vi "vision - Copy.vi"(0 "Image 3":T1(plugin-control)) -> ()   [LabVIEW 2018]
uses:
  Vision info.vi
panel:
  out "cir 2":cluster{"x":dbl, "y":dbl, "r":dbl}[](array[cluster])
  out "cir":cluster{"x":dbl, "y":dbl, "r":dbl}[](array[cluster])
  out "Circles 2":cluster{"x":dbl, "y":dbl, "r":dbl}[](array[cluster])
  out "cube found":bool
  out "Type":enum16{"Z", "I", "O", "S", "L", "J", "T", "N"}(ring)=enum."O"
  out "Discriptor":dbl[](array[numeric])
  out "Image 2":T1(plugin-control)
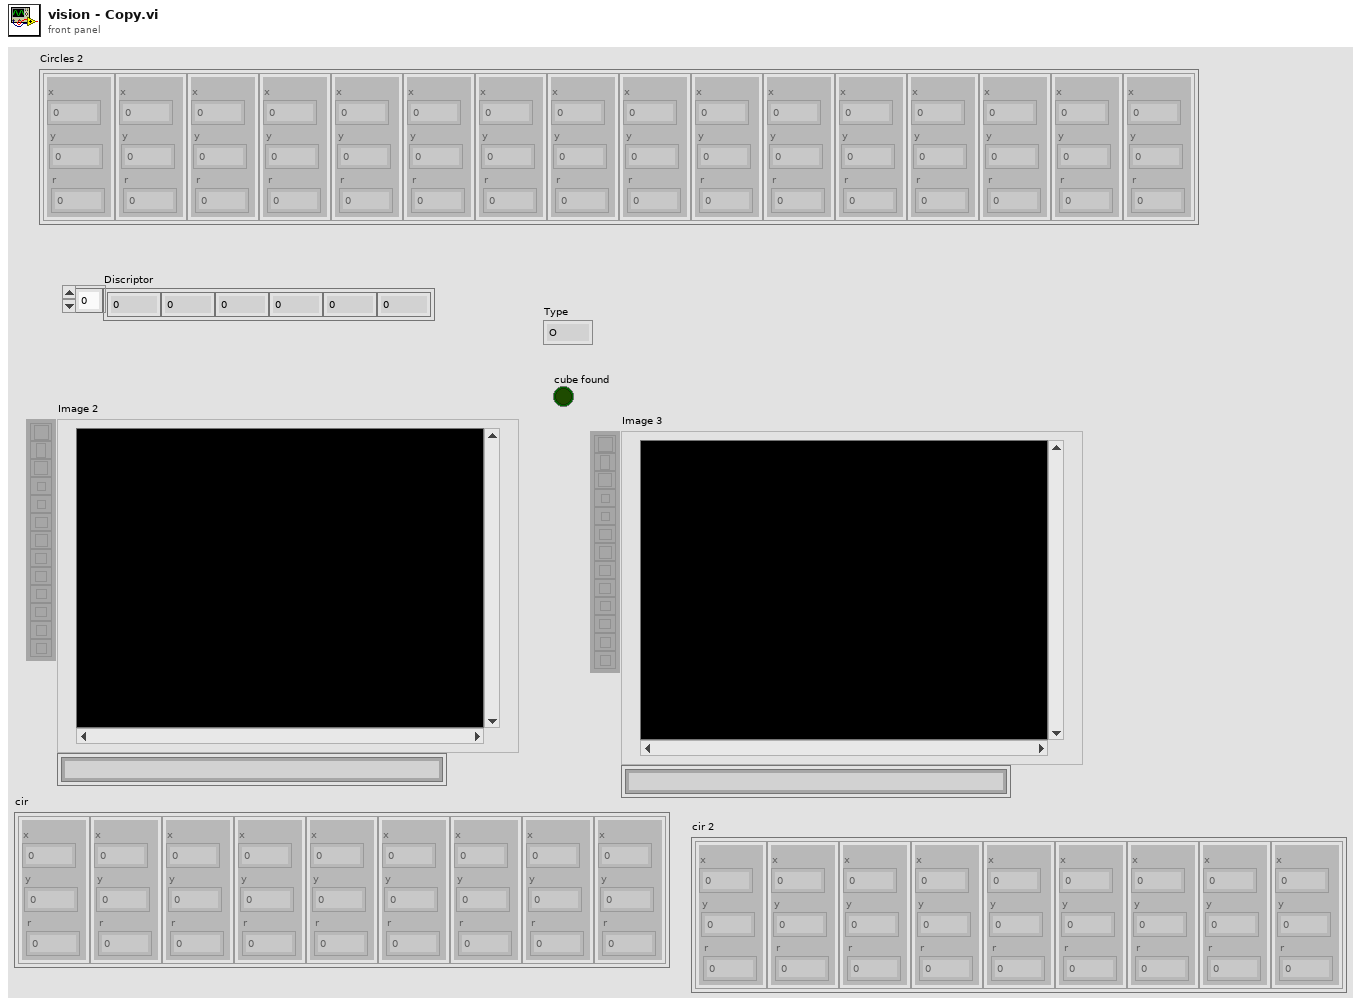
[diagram p1: front panel]
types:
  T1 = typedef "IMAQ Image.ctl" = refnum<image>
  T2 = cluster{"p1":cluster{"x":dbl, "y":dbl}, "p2":cluster{"x":dbl, "y":dbl}}
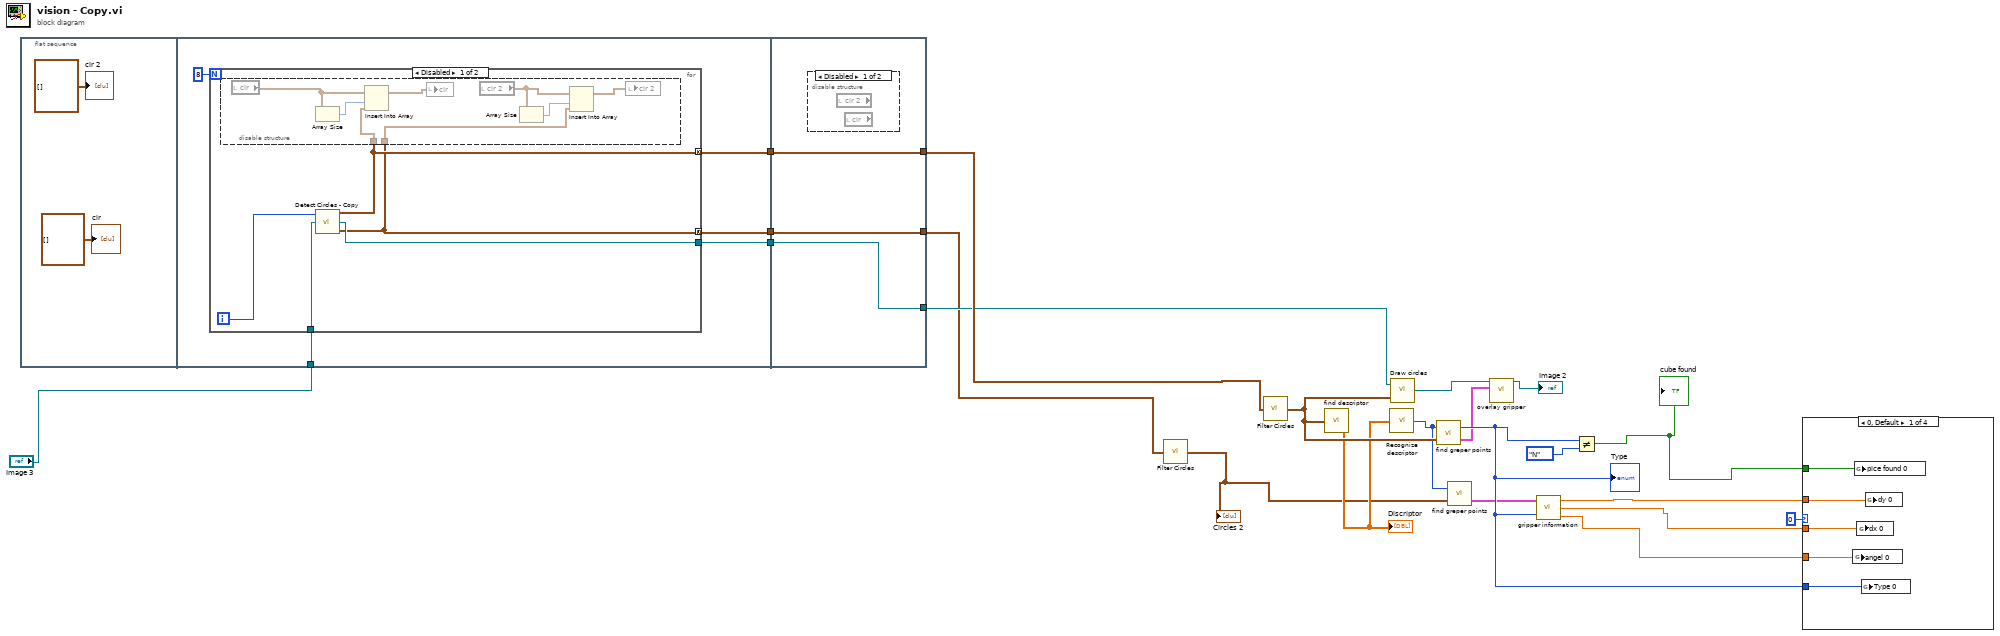
[diagram p0: block diagram]
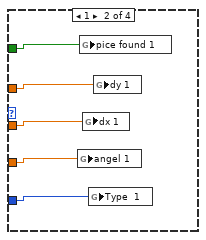
[diagram p4: hidden frame]
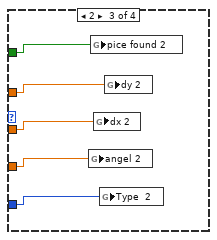
[diagram p5: hidden frame]
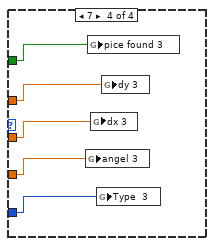
[diagram p6: hidden frame]
diagram:
  n1 = flat-sequence {
    tunnel: "Image 3" -> [w28]
    tunnel: [w27] -> w7
    tunnel: [w26] -> w4
    tunnel: [w25] -> w3
    tunnel: [w44] -> w8
    tunnel: [w43] -> w2
    tunnel: [w45] -> w5
    tunnel: w7 -> [w45]
    tunnel: w4 -> [w44]
    tunnel: w3 -> [w43]
    frame #0 {
      "cir" <- cluster{"x":dbl, "y":dbl, "r":dbl}[] [] ("cir")
      "cir 2" <- cluster{"x":dbl, "y":dbl, "r":dbl}[] [] ("cir")
    }
    frame #1 {
      n2 = for {
        N: 8 -> [_]
        tunnel: w28 -> [w33]
        tunnel: [w32] -> w27
        tunnel: [w31] -> w26 mode=concatenating
        tunnel: [w30] -> w25 mode=concatenating
        i -> [w34]
        n3 = call "Detect Circles - Copy.vi"("Image 3"=w33, "Color Plane"=w34) -> ("Circles 2"=w30:cluster{"x":dbl, "y":dbl, "r":dbl}[], "Image 4"=w32:T1, "Circles"=w31:cluster{"x":dbl, "y":dbl, "r":dbl}[])  [unwired: 1 in]
        n4 = disable-structure shown="Disabled" {
          disable-tunnel: w31 -> [w39 _]
          disable-tunnel: w30 -> [w36 _]
          frame Disabled {
            n5 = local read "cir"() -> (w41:cluster{"x":dbl, "y":dbl, "r":dbl}[])
            n6 = Array Size(array=w41) -> (size(s)=w40:i32)
            n7 = Insert Into Array(array=w41, index=w40, new element=w39) -> (w42:cluster{"x":dbl, "y":dbl, "r":dbl}[])
            n8 = local write "cir"(w42) -> ()
            n9 = local read "cir 2"() -> (w35:cluster{"x":dbl, "y":dbl, "r":dbl}[])
            n10 = Array Size(array=w35) -> (size(s)=w38:i32)
            n11 = Insert Into Array(array=w35, index=w38, new element=w36) -> (w37:cluster{"x":dbl, "y":dbl, "r":dbl}[])
            n12 = local write "cir 2"(w37) -> ()
          }
          frame Enabled {
          }
        }
      }
    }
    frame #2 {
      n13 = disable-structure shown="Disabled" {
        frame Disabled {
          n14 = local read "cir 2"() -> ()  [unwired: 1 out]
          n15 = local read "cir"() -> ()  [unwired: 1 out]
        }
        frame Enabled {
        }
      }
    }
  }
  n16 = call "Filter Circles.vi"("Circles"=w2) -> ("out"=w1:cluster{"x":dbl, "y":dbl, "r":dbl}[])
  "Circles 2" <- w1
  n17 = call "Filter Circles.vi"("Circles"=w8) -> ("out"=w17:cluster{"x":dbl, "y":dbl, "r":dbl}[])
  n18 = call "find descriptor.vi"("Circles"=w17) -> ("d"=w14:dbl[])
  "Discriptor" <- w14
  n19 = call "Recognize descriptor.vi"("Discriptor"=w14) -> ("Type"=w11:enum16{"Z", "I", "O", "S", "L", "J", "T", "N"})
  n20 = call "Draw circles .vi"("Circles"=w17, "Image 3"=w5) -> ("Refnum out"=w13:T1)
  n21 = call "find greper points.vi"("Circles"=w17, "Type  2"=w11) -> ("gripper"=w15:T2, "Type"=w22:enum16{"Z", "I", "O", "S", "L", "J", "T", "N"})
  "Type" <- w22
  n22 = call "find greper points.vi"("Circles"=w1, "Type  2"=w11) -> ("gripper"=w10:T2)  [unwired: 1 out]
  n23 = call "overlay gripper.vi"("gripper"=w15, "Refnum in"=w13) -> ("Refnum out"=→"Image 2":T1)  [unwired: 9 in]
  n24 = call "gripper information.vi"("gripper"=w10, "Type"=w22) -> ("dy"=w19:dbl, "dx"=w20:dbl, "Angel"=w21:dbl)
  n25 = Not Equal?(x=w22, y=enum16{"Z", "I", "O", "S", "L", "J", "T", "N"}."N") -> (x != y?=w18:bool)
  "cube found" <- w18
  n26 = case shown="0, Default" 0 ("Color Plane") {
    tunnel: w18 -> [w50 w55 w60 w65]
    tunnel: w19 -> [w49 w54 w59 w64]
    tunnel: w20 -> [w48 w53 w58 w63]
    tunnel: w21 -> [w47 w52 w57 w62]
    tunnel: w22 -> [w46 w51 w56 w61]
    frame 0, Default {
      n27 = global write "Vision info.vi" "angel 0"(w47) -> ()
      n28 = global write "Vision info.vi" "pice found 0"(w50) -> ()
      n29 = global write "Vision info.vi" "dx 0"(w48) -> ()
      n30 = global write "Vision info.vi" "Type 0"(w46) -> ()
      n31 = global write "Vision info.vi" "dy 0"(w49) -> ()
    }
    frame 1 {
      n32 = global write "Vision info.vi" "angel 1"(w52) -> ()
      n33 = global write "Vision info.vi" "pice found 1"(w55) -> ()
      n34 = global write "Vision info.vi" "dx 1"(w53) -> ()
      n35 = global write "Vision info.vi" "Type  1"(w51) -> ()
      n36 = global write "Vision info.vi" "dy 1"(w54) -> ()
    }
    frame 2 {
      n37 = global write "Vision info.vi" "angel 2"(w57) -> ()
      n38 = global write "Vision info.vi" "pice found 2"(w60) -> ()
      n39 = global write "Vision info.vi" "dx 2"(w58) -> ()
      n40 = global write "Vision info.vi" "Type  2"(w56) -> ()
      n41 = global write "Vision info.vi" "dy 2"(w59) -> ()
    }
    frame 7 {
      n42 = global write "Vision info.vi" "angel 3"(w62) -> ()
      n43 = global write "Vision info.vi" "pice found 3"(w65) -> ()
      n44 = global write "Vision info.vi" "dx 3"(w63) -> ()
      n45 = global write "Vision info.vi" "Type  3"(w61) -> ()
      n46 = global write "Vision info.vi" "dy 3"(w64) -> ()
    }
  }
